vi "Get Message Type.vi"(10 "error in (no error)":errorcluster, 11 "JSON":string) -> (0 "<JSON>":string[](array[string]) caption="<JSON>Elements", 1 "Message Codes":T1=1 items=["HELLO"=1, "WELCOME"=2, "ABORT"=3, "GOODBYE"=6, "ERROR"=8, "PUBLISH"=16, "PUBLISHED"=17, "SUBSCRIBE"=32, "SUBSCRIBED"=33, "UNSUBSCRIBE"=34, "UNSUBSCRIBED"=35, "EVENT"=36, "CALL"=48, "RESULT"=59, "REGISTER"=64, "REGISTERED"=65, "UNREGISTER"=66, "UNREGISTERED"=67, "INVOCATION"=68, "YIELD"=70], 2 "error out":errorcluster)   [LabVIEW 2020, in "WAMP Client.lvclass"]
uses:
  <userlib>/lvwamp/WAMP Client/WAMP Client.lvclass
  <userlib>/lvwamp/MessageCodes.ctl
  8f5a4108-e887-cc40-a403-622f77475334.vi
  <vilib>/JDP Science/JSONtext/JSON text to Variant.vi
  <vilib>/JDP Science/JSONtext/LVClass Serializer/JSONtext LVClass Serializer.lvclass
  <vilib>/JDP Science/JSONtext/JSONtext.lvlib
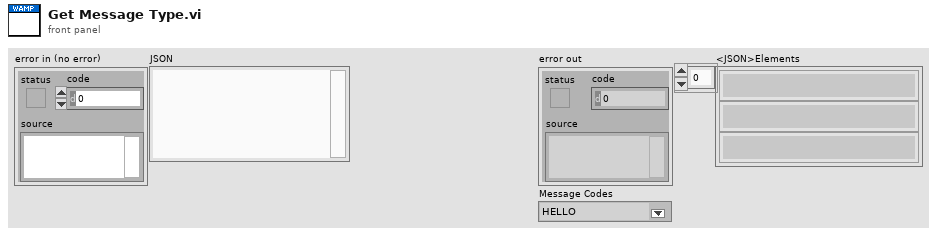
[diagram p1: front panel]
types:
  T1 = typedef "WAMP Client.lvclass/MessageCodes.ctl" = u16
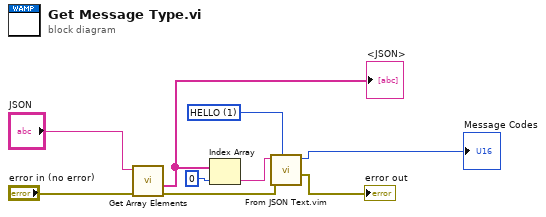
[diagram p0: block diagram]
diagram:
  w3 = T1 1 items=["HELLO"=1, "WELCOME"=2, "ABORT"=3, "GOODBYE"=6, "ERROR"=8, "PUBLISH"=16, "PUBLISHED"=17, "SUBSCRIBE"=32, "SUBSCRIBED"=33, "UNSUBSCRIBE"=34, "UNSUBSCRIBED"=35, "EVENT"=36, "CALL"=48, "RESULT"=59, "REGISTER"=64, "REGISTERED"=65, "UNREGISTER"=66, "UNREGISTERED"=67, "INVOCATION"=68, "YIELD"=70] ("Message Codes")
  n1 = call <vilib>:"Get Array Elements.vi"("error in (no error)"="error in (no error)", "JSON"="JSON") -> ("error out"=w4:errorcluster, "<JSON>"=w9:string[])  [unwired: 7 in, 1 out]
  "<JSON>" <- w9
  n2 = Index Array(array=w9, index=0) -> (element=w5:string)
  n3 = call "From JSON Text.vim"("Data Type and Default Value"=w3, "error in (no error)"=w4, "JSON"=w5) -> ("error out"=→"error out":errorcluster, "Data out"=→"Message Codes":T1)  [unwired: 7 in]
